vi "Build.vi"(7 "conversion descriptor":T1 {"conversions"."converted descriptor"."buffer offset" format="%d bytes"; "conversions"."unconverted descriptor"."buffer offset" format="%d bytes"}, 8 "error in (no error)":errorcluster, 9 "converted Buffer":refnum<class "Buffer.lvclass">, 10 "unconverted Buffer":refnum<class "Buffer.lvclass">, 11 "Buffer Converter in":refnum<class "Buffer Converter.lvclass">) -> (0 "error out":errorcluster, 3 "Buffer Converter out":refnum<class "Buffer Converter.lvclass">)   [LabVIEW 2017, in "DSF Core.lvlib" / "Buffer Converter.lvclass"]
uses:
  Buffer Converter.lvclass
  Buffer/Buffer.lvclass
  Type Conversion Descriptor.ctl
  Type Conversion.ctl
  Channel Descriptor.ctl
  DSF Configuration API/Public/Controls/DSF Data Type.ctl
  Buffer Converter.lvclass/Buffer Converter.ctl
  Buffer/Buffer.lvclass/Buffer.ctl
  Convert String Type Subset.vi
  Shared/VIs/Sizeof 1D.vi
  Shared/VIs/Sizeof.vi
  Buffer/Read Buffer String.vi
  Buffer/Write Buffer String.vi
  DSF Core.lvlib
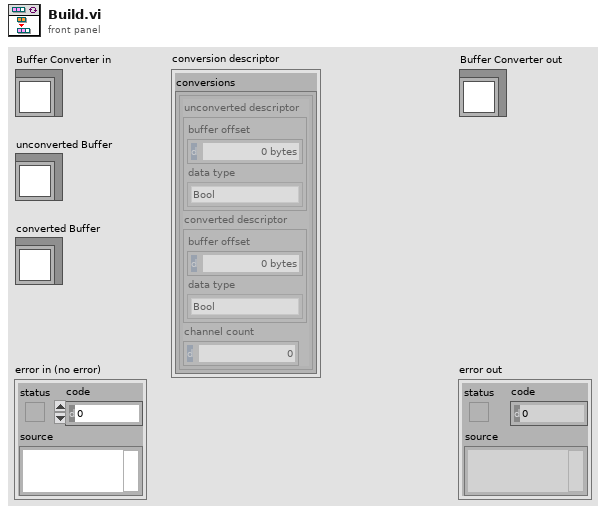
[diagram p1: front panel]
types:
  T1 = typedef "DSF Core.lvlib/Buffer Converter.lvclass/Type Conversion Descriptor.ctl" = cluster{"conversions":T2[]}
  T2 = typedef "DSF Core.lvlib/Buffer Converter.lvclass/Type Conversion.ctl" = cluster{"unconverted descriptor":T3, "converted descriptor":T3, "channel count":u64}
  T3 = typedef "DSF Core.lvlib/Buffer.lvclass/Channel Descriptor.ctl" = cluster{"buffer offset":u64, "data type":T4}
  T4 = typedef "DSF Core.lvlib/DSF Data Type.ctl" = enum8{"Bool", "SGL", "DBL", "I8", "I16", "I32", "I64", "U8", "U16", "U32", "U64"}
  T5 = enum16{"big-endian, network order", "native, host order", "little-endian"}
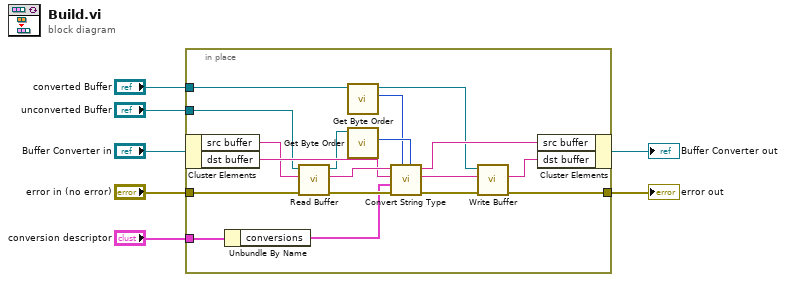
[diagram p0: block diagram]
diagram:
  n1 = in-place {
    in-place-border: "unconverted Buffer" -> [w12]
    in-place-border: "converted Buffer" -> [w16]
    in-place-border: [w24] -> w5
    in-place-border: "error in (no error)" -> [w22]
    in-place-border: "conversion descriptor" -> [w17]
    n2 = in-place-cluster #1("Buffer Converter in") -> ("src buffer"=w14:string, "dst buffer"=w20:string)
    n3 = Unbundle By Name(w17) -> ("conversions"=w9:T2[])
    n4 = call-poly "Read Buffer.vi"("error in (no error)"=w22, "dst string in"=w14, "Buffer in"=w12) -> ("error out"=w23:errorcluster, "dst string out"=w21:string, "Buffer out"=w13:refnum<class "Buffer.lvclass">)  [unwired: 5 in, 1 out]
    n5 = call "Get Byte Order.vi"("Buffer in"=w16) -> ("byte order"=w11:T5, "Buffer out"=w10:refnum<class "Buffer.lvclass">)  [unwired: 9 in]
    n6 = call "Get Byte Order.vi"("Buffer in"=w13) -> ("byte order"=w15:T5)  [unwired: 9 in, 1 out]
    n7 = call "Convert String Type.vi"("src byte order"=w15, "dst byte order"=w11, "error in (no error)"=w23, "conversions"=w9, "dst buffer in"=w20, "src buffer in"=w21) -> ("error out"=w25:errorcluster, "dst buffer out"=w18:string, "src buffer out"=w19:string)  [unwired: 3 in]
    n8 = call-poly "Write Buffer.vi"("error in (no error)"=w25, "src string in"=w18, "Buffer in"=w10) -> ("error out"=w24:errorcluster, "src string out"=w8:string)  [unwired: 5 in, 2 out]
    n9 = in-place-cluster #1("src buffer"=w19, "dst buffer"=w8) -> (→"Buffer Converter out":refnum<class "Buffer Converter.lvclass">)
  }
  "error out" <- w5
